vi "normal_Flow.vi"(8 "error in":errorcluster, 11 "VISA resource name":refnum<visa-resource-name>="ASRL2::INSTR") -> (0 "error out":errorcluster, 3 "VISA resource out":refnum<visa-resource-name>="ASRL2::INSTR")   [LabVIEW 2010]
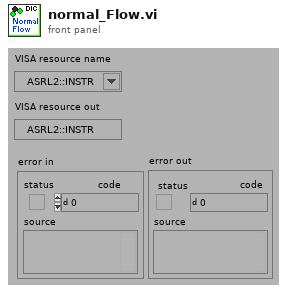
[diagram p1: front panel]
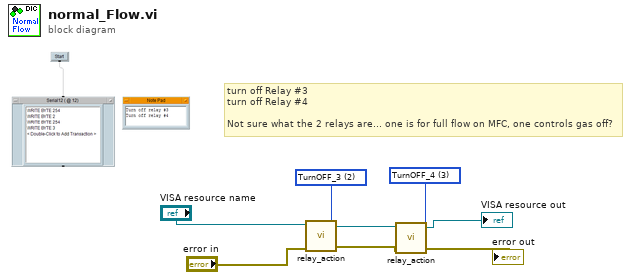
[diagram p0: block diagram]
diagram:
  w3 = u8 3 items=["TurnON_1"=8, "TurnON_PUMP"=9, "TurnON_3"=10, "TurnON_4"=11, "CLOSE DUMP OFF_1"=0, "TurnOFF_PUMP"=1, "TurnOFF_3"=2, "TurnOFF_4"=3, "OpenAll"=30, "CloseAllRelay"=29] ("Action 2")
  w6 = u8 2 items=["TurnON_1"=8, "TurnON_PUMP"=9, "TurnON_3"=10, "TurnON_4"=11, "CLOSE DUMP OFF_1"=0, "TurnOFF_PUMP"=1, "TurnOFF_3"=2, "TurnOFF_4"=3, "OpenAll"=30, "CloseAllRelay"=29] ("Action")
  # "turn off Relay #3\nturn off Relay #4\n\nNot sure what the 2 relays are... one is for full flow on MFC, one controls gas off?"
  n1 = call "relay_action.vi"("VISA resource in"="VISA resource name", "Action"=w6, "error in"="error in") -> ("VISA resource out"=w5:refnum<visa-resource-name>, "error out"=w4:errorcluster)  [unwired: 4 in]
  n2 = call "relay_action.vi"("VISA resource in"=w5, "Action"=w3, "error in"=w4) -> ("VISA resource out"=→"VISA resource out":refnum<visa-resource-name>, "error out"=→"error out":errorcluster)  [unwired: 4 in]
